vi "Image In Clipoboard to PNG File.vi"(8 "error in (no error)":errorcluster, 11 "Image Path":path) -> (0 "error out":errorcluster)   [LabVIEW 2017, in "Error Dialog w Copy to Clipboard.lvlib"]
uses:
  Error Dialog w Copy to Clipboard.lvlib
  System.Windows.Forms
  System.Drawing
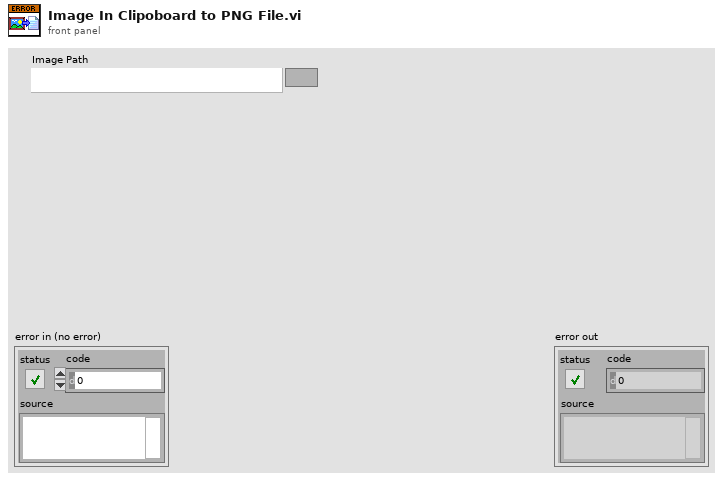
[diagram p1: front panel]
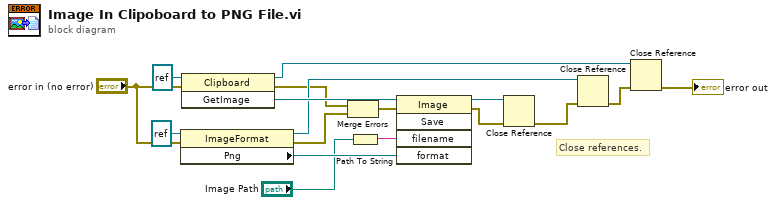
[diagram p0: block diagram]
diagram:
  # "Close references."
  n1 = property class="ImageFormat"(reference=refnum<k24> refnum, error in="error in (no error)") -> (reference out=w11:refnum<k24>, error out=w7:errorcluster, "Png"=w17:refnum<k24>)
  n2 = invoke class="Clipboard" method="GetImage"(reference=refnum<k24> refnum, error in="error in (no error)") -> (reference out=w9:refnum<k24>, error out=w4:errorcluster, "GetImage"=w15:refnum<k24>)  [unwired: 1 in]
  n3 = Merge Errors(w4, w7) -> (w5:errorcluster)
  n4 = Path To String(path="Image Path") -> (string=w16:string)
  n5 = invoke class="Image" method="Save"(reference=w15, error in=w5, "filename"=w16, "format"=w17) -> (reference out=w13:refnum<k24>, error out=w14:errorcluster)  [unwired: 1 in, 3 out]
  n6 = Close Reference(reference=w13, error in (no error)=w14) -> (error out=w12:errorcluster)
  n7 = Close Reference(reference=w11, error in (no error)=w12) -> (error out=w10:errorcluster)
  n8 = Close Reference(reference=w9, error in (no error)=w10) -> (error out=→"error out":errorcluster)
